vi "Exercice 3.vi"() -> ()   [LabVIEW 2019]
uses:
  <vilib>/myRIO/Instrument Drivers/Onboard Devices/Accelerometer/typedefs/Accelerometer Reference.ctl
  <vilib>/myRIO/Common/Instrument Driver Framework/Utilities/typedefs/myRIO Generic Hardware Reference.ctl
  <vilib>/myRIO/Common/Instrument Driver Framework/Utilities/typedefs/Hardware Version Enum.ctl
  <vilib>/myRIO/Common/Instrument Driver Framework/Utilities/typedefs/myRIO v1.0 Reference.ctl
  <vilib>/myRIO/Common/Instrument Driver Framework/Utilities/typedefs/Generic FPGA Reference.ctl
  <vilib>/myRIO/Common/Instrument Driver Framework/myRIO v1.0/Accelerometer/typedefs/Accelerometer Channels List.ctl
  <vilib>/myRIO/Common/Instrument Driver Framework/myRIO v1.0/Accelerometer/typedefs/Accelerometer Channels Enum.ctl
  <vilib>/userDefined/High Color/nirio_resource_hc.ctl
  <vilib>/myRIO/Instrument Drivers/Onboard IO/DIO/typedefs/DIO Reference.ctl
  <vilib>/myRIO/Common/Instrument Driver Framework/myRIO v1.0/DIO/typedefs/DIO Channels List.ctl
  <vilib>/myRIO/Common/Instrument Driver Framework/myRIO v1.0/DIO/typedefs/DIO Channels Enum.ctl
  <vilib>/myRIO/Common/Instrument Driver Framework/Utilities/vis/Is FPGA Ref Available.vi
  <vilib>/myRIO/Common/Instrument Driver Framework/myRIO v1.0/DIO/vis/myRIO v1.1 Open DIO.vi
  <vilib>/myRIO/Instrument Drivers/Onboard IO/DIO/vis/Read.vi
  <vilib>/myRIO/Common/Instrument Driver Framework/myRIO v1.0/Accelerometer/vis/myRIO v1.1 Open Accelerometer.vi
  <vilib>/myRIO/Instrument Drivers/Onboard Devices/Accelerometer/vis/Read.vi
  <vilib>/myRIO/Instrument Drivers/Onboard IO/DIO/vis/Write.vi
  <vilib>/myRIO/Common/Instrument Driver Framework/Utilities/vis/Validate Channels.vi
  <vilib>/myRIO/Common/Instrument Driver Framework/myRIO v1.0/DIO/vis/myRIO v1.0 Reserve DIO.vi
  <vilib>/myRIO/Common/Instrument Driver Framework/myRIO v1.0/Accelerometer/vis/myRIO v1.0 Reserve Accelerometer.vi
  <vilib>/myRIO/Common/Instrument Driver Framework/myRIO v1.0/Resource Manager/vis/myRIO v1.0 Reserve Channel List.vi
  <vilib>/myRIO/Common/Instrument Driver Framework/myRIO v1.0/DIO/vis/myRIO v1.0 Build MUX Configuration DIO.vi
  <vilib>/myRIO/Common/Instrument Driver Framework/myRIO v1.0/Accelerometer/vis/myRIO v1.0 Build MUX Configuration Accelerometer.vi
  <vilib>/myRIO/Common/Instrument Driver Framework/myRIO v1.0/Resource Manager/vis/myRIO v1.0 Reserve Channel.vi
  <vilib>/myRIO/Common/Instrument Driver Framework/myRIO v1.0/Resource Manager/vis/myRIO v1.0 Unreserve Channel.vi
  <vilib>/myRIO/Common/Instrument Driver Framework/myRIO v1.0/Resource Manager/vis/myRIO v1.0 Create Configuration List.vi
  <vilib>/myRIO/Common/Instrument Driver Framework/myRIO v1.0/Resource Manager/vis/myRIO v1.0 Build Mutex Name.vi
  <vilib>/Utility/VariantDataType/GetNumericInfo.vi
  <vilib>/Utility/error.llb/Error Cluster From Error Code.vi
  <vilib>/myRIO/Common/Instrument Driver Framework/myRIO v1.0/myRIO v1.1 Open.vi
  <vilib>/myRIO/Common/Instrument Driver Framework/myRIO v1.0/Accelerometer/vis/myRIO v1.0 Get Scaling Constant Accelerometer.vi
  <vilib>/myRIO/Common/Instrument Driver Framework/Utilities/vis/IO Manager.vi
  <vilib>/myRIO/Common/Instrument Driver Framework/Utilities/vis/Configuration Manager.vi
  <vilib>/myRIO/Common/Instrument Driver Framework/myRIO v1.0/myRIO v1.0 Close.vi
  <vilib>/myRIO/Common/Instrument Driver Framework/myRIO v1.0/Accelerometer/vis/myRIO v1.0 Read Accelerometer.vi
  <vilib>/myRIO/Common/Instrument Driver Framework/myRIO v1.0/Resource Manager/vis/myRIO v1.0 Configure IO.vi
  <vilib>/myRIO/Common/Instrument Driver Framework/myRIO v1.0/DIO/vis/myRIO v1.0 Read DIO.vi
  <vilib>/myRIO/Common/Instrument Driver Framework/myRIO v1.0/DIO/vis/myRIO v1.0 Write DIO.vi
  <vilib>/myRIO/Express VI/Onboard Devices/Accelerometer/Accelerometer Express VI.xnode
  <vilib>/myRIO/Instrument Drivers/Onboard Devices/Accelerometer/vis/myRIO Accelerometer Open.xnode
  <vilib>/myRIO/Express VI/Onboard Devices/Button/Button Express VI.xnode
  <vilib>/myRIO/Instrument Drivers/Onboard IO/DIO/vis/myRIO DIO Open.xnode
  <vilib>/myRIO/Express VI/Onboard Devices/LED/LED Express VI.xnode
  <vilib>/myRIO/Instrument Drivers/Onboard Devices/Accelerometer/Accelerometer.lvlib
  <vilib>/myRIO/Instrument Drivers/Onboard IO/DIO/DIO.lvlib
panel:
  in  "stop":bool
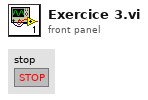
[diagram p1: front panel]
types:
  T1 = typedef "DIO.lvlib/DIO Reference.ctl" = cluster{"myRIO Reference":T2, "DIO Channels List":T6}
  T2 = typedef "myRIO Generic Hardware Reference.ctl" = cluster{"myRIO Model":T3, "myRIO Hardware Reference":T4}
  T3 = typedef "Hardware Version Enum.ctl" = enum16{"Unknown", "myRIO-1900", "myRIO-1950", "roboRIO", "NI ELVIS RIO CM", "ELVIS III"}
  T4 = typedef "myRIO v1.0 Reference.ctl" = cluster{"Generic FPGA Reference":T5, "Allow multiple opens":bool}
  T5 = typedef "Generic FPGA Reference.ctl" = refnum<k20>
  T6 = typedef "DIO Channels List.ctl" = T7[]
  T7 = typedef "DIO Channels Enum.ctl" = enum16{"Not Connected", "C/DIO0", "C/DIO1", "C/DIO2", "C/DIO3", "C/DIO4", "C/DIO5", "C/DIO6", "C/DIO7", "A/DIO0", "A/DIO1", "A/DIO2", "A/DIO3", "A/DIO4", "A/DIO5", "A/DIO6", "A/DIO7", "A/DIO8", "A/DIO9", "A/DIO10", "A/DIO11", "A/DIO12", "A/DIO13", "A/DIO14", "A/DIO15", "A/DIO16", "A/DIO17", "A/DIO18", "A/DIO19", "B/DIO0", "B/DIO1", "B/DIO2", "B/DIO3", "B/DIO4", "B/DIO5", "B/DIO6", "B/DIO7", "B/DIO8", "B/DIO9", "B/DIO10", "B/DIO11", "B/DIO12", "B/DIO13", "B/DIO14", "B/DIO15", "B/DIO16", "B/DIO17", "B/DIO18", "B/DIO19", "LED0", "LED1", "LED2", "LED3", "Button0", "DIO/DIO0", "DIO/DIO1", "DIO/DIO2", "DIO/DIO3", "DIO/DIO4", "DIO/DIO5", "DIO/DIO6", "DIO/DIO7", "DIO/DIO8", "DIO/DIO9", "SPI/CS0", "SPI/CS1", "SPI/CS2", "SPI/CS3", "LED RADIO (Green)", "LED RADIO (Red)", "LED COMM (Green)", "LED COMM (Red)", "LED MODE (Green)", "LED MODE (Red)"}
  T8 = typedef "nirio_resource_hc.ctl" = tag
  T9 = typedef "Accelerometer.lvlib/Accelerometer Reference.ctl" = cluster{"myRIO Reference":T2, "Accelerometer Channels List":T10, "LSB Weight":dbl}
  T10 = typedef "Accelerometer Channels List.ctl" = T11[]
  T11 = typedef "Accelerometer Channels Enum.ctl" = enum16{"Not Connected", "X-Axis", "Y-Axis", "Z-Axis"}
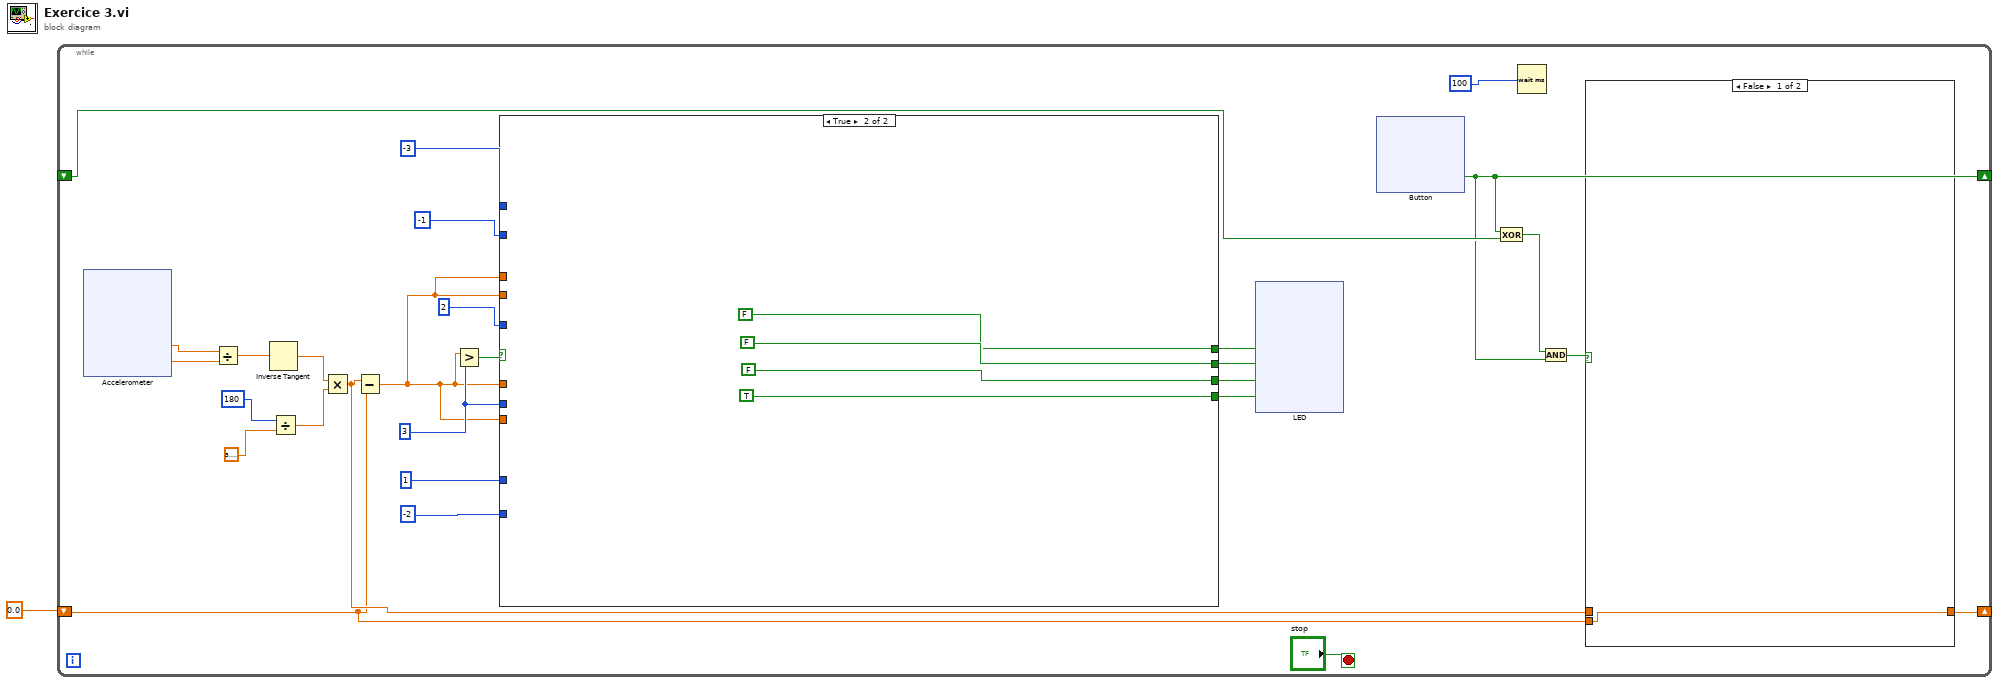
[diagram p0: block diagram]
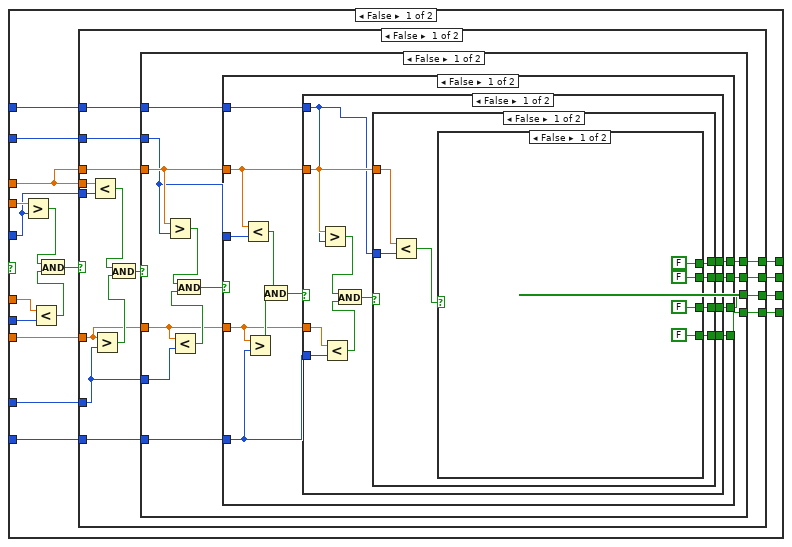
[diagram p3: hidden frame]
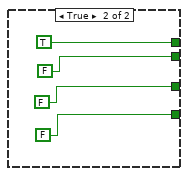
[diagram p4: hidden frame]
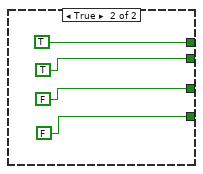
[diagram p5: hidden frame]
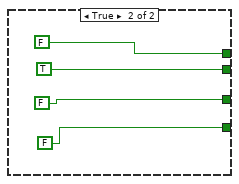
[diagram p6: hidden frame]
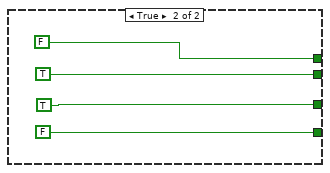
[diagram p7: hidden frame]
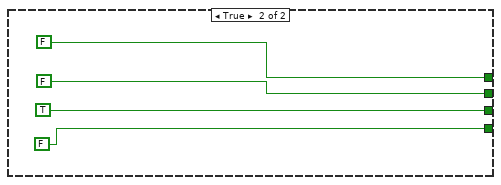
[diagram p8: hidden frame]
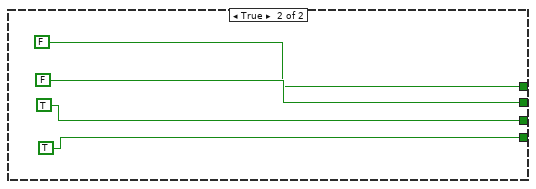
[diagram p9: hidden frame]
diagram:
  n1 = while {
    shift-right: [w11] -> _
    shift-left: _ -> [w15]
    shift-right: [w12] -> _
    shift-left: 0.0 -> [w2]
    stop <- "stop" stop-if-true
    w7 = 3
    n2 = xnode "Accelerometer"() -> ("Y"=w29:dbl, "Z"=w28:dbl)  [unwired: 1 in, 2 out]
    n3 = Divide(x=w29, y=w28) -> (x/y=w27:dbl)
    n4 = Inverse Tangent(1:w27) -> (0:w23:dbl)
    n5 = Divide(x=180, y=3.141592653589793) -> (x/y=w24:dbl)
    n6 = Multiply(x=w23, y=w24) -> (x*y=w3:dbl)
    n7 = Subtract(x=w3, y=w2) -> (x-y=w5:dbl)
    n8 = Greater?(x=w5, y=w7) -> (0:w22:bool)
    n9 = case shown="True" w22 {
      tunnel: [w76 TRUE ("3")] -> w21
      tunnel: 2 -> [w75 _]
      tunnel: w5 -> [w83 _]
      tunnel: w5 -> [w82 _]
      tunnel: w7 -> [w81 _]
      tunnel: [w77 FALSE ("2")] -> w20
      tunnel: w5 -> [w72 _]
      tunnel: w5 -> [w74 _]
      tunnel: 1 -> [w73 _]
      tunnel: -1 -> [w71 _]
      tunnel: [w70 FALSE ("1")] -> w19
      tunnel: -2 -> [w69 _]
      tunnel: -3 -> [w68 _]
      tunnel: [w67 FALSE ("0")] -> w18
      frame False {
        n10 = Greater?(x=w83, y=w75) -> (0:w79:bool)
        n11 = Less?(x=w82, y=w81) -> (x < y?=w78:bool)
        n12 = And(x=w79, y=w78) -> (x .and. y?=w80:bool)
        n13 = case shown="False" w80 {
          tunnel: [w93 TRUE ("2")] -> w77
          tunnel: [w84 TRUE ("3")] -> w76
          tunnel: w72 -> [w98 _]
          tunnel: w75 -> [w97 _]
          tunnel: w74 -> [w92 _]
          tunnel: w73 -> [w91 _]
          tunnel: w72 -> [w90 _]
          tunnel: w71 -> [w89 _]
          tunnel: [w88 FALSE ("1")] -> w70
          tunnel: w69 -> [w87 _]
          tunnel: w68 -> [w86 _]
          tunnel: [w85 FALSE ("0")] -> w67
          frame False {
            n14 = Less?(x=w98, y=w97) -> (x < y?=w95:bool)
            n15 = Greater?(x=w92, y=w91) -> (0:w94:bool)
            n16 = And(x=w95, y=w94) -> (x .and. y?=w96:bool)
            n17 = case shown="False" w96 {
              tunnel: [w106 TRUE ("2")] -> w93
              tunnel: w92 -> [w105 _]
              tunnel: w91 -> [w111 _]
              tunnel: w90 -> [w103 _]
              tunnel: w89 -> [w102 _]
              tunnel: [w107 FALSE ("1")] -> w88
              tunnel: w87 -> [w104 _]
              tunnel: w86 -> [w101 _]
              tunnel: [w100 FALSE ("0")] -> w85
              tunnel: [w99 FALSE ("3")] -> w84
              frame False {
                n18 = Greater?(x=w103, y=w102) -> (0:w109:bool)
                n19 = Less?(x=w105, y=w111) -> (x < y?=w108:bool)
                n20 = And(x=w109, y=w108) -> (x .and. y?=w110:bool)
                n21 = case shown="False" w110 {
                  tunnel: [w119 TRUE ("1")] -> w107
                  tunnel: [w113 TRUE ("2")] -> w106
                  tunnel: w105 -> [w118 _]
                  tunnel: w104 -> [w117 _]
                  tunnel: w103 -> [w115 _]
                  tunnel: w102 -> [w123 _]
                  tunnel: w101 -> [w116 _]
                  tunnel: [w114 FALSE ("0")] -> w100
                  tunnel: [w112 FALSE ("3")] -> w99
                  frame False {
                    n22 = Less?(x=w115, y=w123) -> (x < y?=w121:bool)
                    n23 = Greater?(x=w118, y=w117) -> (0:w120:bool)
                    n24 = And(x=w121, y=w120) -> (x .and. y?=w122:bool)
                    n25 = case shown="False" w122 {
                      tunnel: [w128 TRUE ("1")] -> w119
                      tunnel: w118 -> [w134 _]
                      tunnel: w117 -> [w133 _]
                      tunnel: w116 -> [w126 _]
                      tunnel: w115 -> [w127 _]
                      tunnel: [w129 FALSE ("0")] -> w114
                      tunnel: [w124 FALSE ("2")] -> w113
                      tunnel: [w125 FALSE ("3")] -> w112
                      frame False {
                        n26 = Greater?(x=w127, y=w126) -> (0:w130:bool)
                        n27 = Less?(x=w134, y=w133) -> (x < y?=w131:bool)
                        n28 = And(x=w130, y=w131) -> (x .and. y?=w132:bool)
                        n29 = case shown="False" w132 {
                          tunnel: [w138 TRUE ("0")] -> w129
                          tunnel: [w137 TRUE ("1")] -> w128
                          tunnel: w127 -> [w141 _]
                          tunnel: w126 -> [w140 _]
                          tunnel: [w135 FALSE ("3")] -> w125
                          tunnel: [w136 FALSE ("2")] -> w124
                          frame False {
                            n30 = Less?(x=w141, y=w140) -> (x < y?=w139:bool)
                            n31 = case shown="False" w139 {
                              tunnel: [FALSE ("0") TRUE ("0")] -> w138
                              tunnel: [FALSE ("1") FALSE ("1")] -> w137
                              tunnel: [FALSE ("2") FALSE ("2")] -> w136
                              tunnel: [FALSE ("3") FALSE ("3")] -> w135
                              frame False {
                              }
                              frame True {
                              }
                            }
                          }
                          frame True {
                          }
                        }
                      }
                      frame True {
                      }
                    }
                  }
                  frame True {
                  }
                }
              }
              frame True {
              }
            }
          }
          frame True {
          }
        }
      }
      frame True {
      }
    }
    n32 = xnode "LED"("0"=w18, "1"=w19, "2"=w20, "3"=w21) -> ()  [unwired: 1 in, 1 out]
    n33 = xnode "Button"() -> ("Value"=w11:bool)  [unwired: 1 in, 1 out]
    n34 = Exclusive Or(1:w15, 2:w11) -> (0:w13:bool)
    n35 = Wait (ms)(milliseconds to wait=100) -> ()  [unwired: 1 out]
    n36 = And(x=w13, y=w11) -> (x .and. y?=w14:bool)
    n37 = case shown="False" w14 {
      tunnel: w3 -> [_ w31]
      tunnel: [w30 w31] -> w12
      tunnel: w2 -> [w30 _]
      frame False {
      }
      frame True {
      }
    }
  }
